vi "_Parse Text.vi"(11 "Text":string) -> (2 "Tokens":T1[](array[typedef]), 3 "Lines":string[](array[string]))   [LabVIEW 2017, in "LabVIEW-Config.lvlib" / "LabVIEW-Config.lvclass"]
uses:
  LabVIEW-Config.lvclass
  LineToken.ctl
  <userlib>/_NEVSTOP/Communicable State Machine(CSM)/Communicable State Machine.lvlib
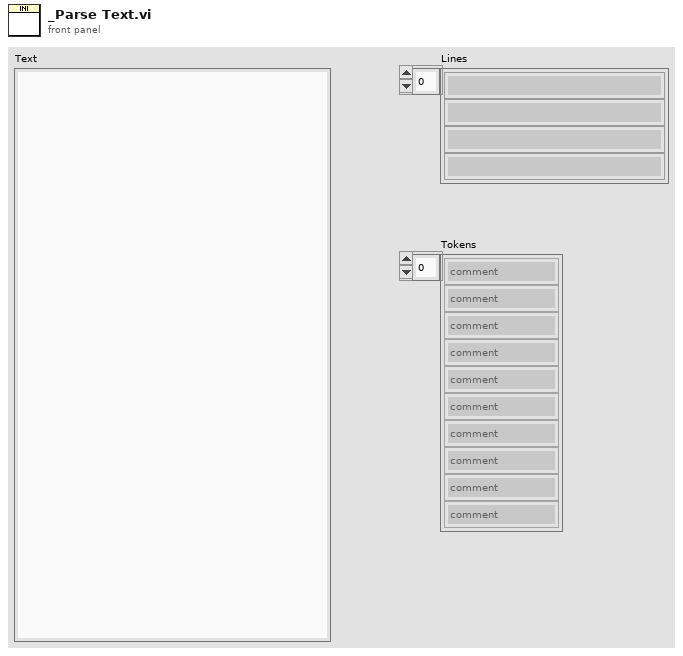
[diagram p1: front panel]
types:
  T1 = typedef "LabVIEW-Config.lvlib/LabVIEW-Config.lvclass/LineToken.ctl" = enum8{"comment", "section", "key", "more"}
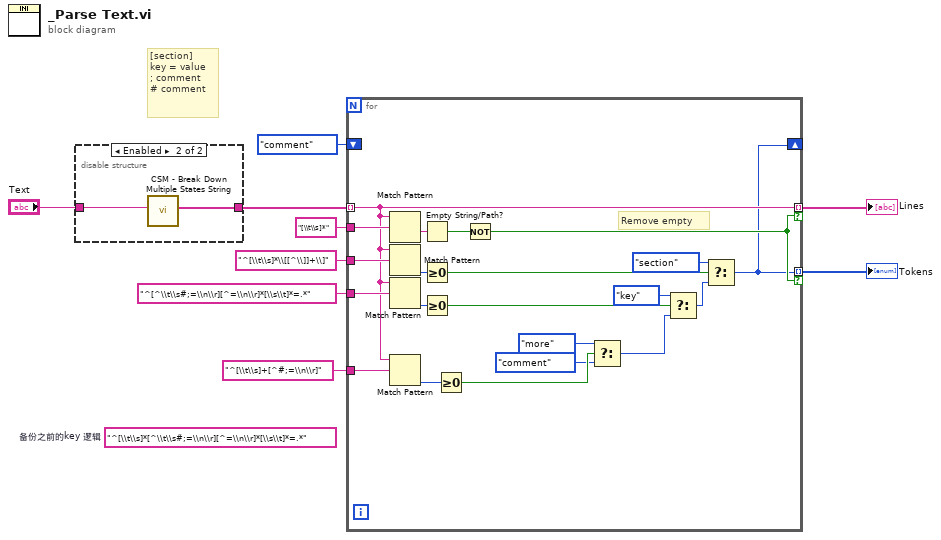
[diagram p0: block diagram]
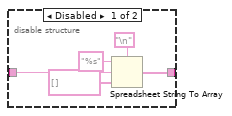
[diagram p2: hidden frame]
diagram:
  (unwired) "^[\\t\\s]*[^\\t\\s#;=\\n\\r][^=\\n\\r]*[\\s\\t]*=.*"  # 备份之前的key 逻辑
  # "[section]\nkey = value\n; comment\n# comment"
  n1 = disable-structure shown="Enabled" {
    disable-tunnel: [w14 w16] -> w7
    disable-tunnel: "Text" -> [w10 w15]
    frame Disabled {
      n2 = Spreadsheet String To Array(delimiter (Tab)="\n" ("Line Feed Constant"), format string="%s", spreadsheet string=w10, array type (2D Dbl)=string[] []) -> (array=w14:string[])
    }
    frame Enabled {
      n3 = call <userlib>:"CSM - Break Down Multiple States String.vi"("States"=w15) -> ("Multiple States"=w16:string[])  [unwired: 10 in]
    }
  }
  n4 = for {
    tunnel: w7 -> [w22] mode=indexing
    tunnel: "^[\\t\\s]*\\[[^\\]]+\\]" ("regular expression") -> [w37]
    tunnel: [w17] -> w2 mode=indexing if=w30
    tunnel: "^[^\\t\\s#;=\\n\\r][^=\\n\\r]*[\\s\\t]*=.*" ("regular expression") -> [w32]
    tunnel: "[\\t\\s]*" ("regular expression") -> [w35]
    tunnel: [w22] -> w6 mode=indexing if=w30
    tunnel: "^[\\t\\s]+[^#;=\\n\\r]" ("regular expression") -> [w23]
    shift-right: [w17] -> _
    shift-left: LineToken."comment" ("Token") -> [_]
    # "Remove empty"
    n5 = Match Pattern(string=w22, regular expression=w35) -> (after substring=w36:string)  [unwired: 1 in, 3 out]
    n6 = Match Pattern(string=w22, regular expression=w37) -> (offset past match=w34:i32)  [unwired: 1 in, 3 out]
    n7 = Match Pattern(string=w22, regular expression=w32) -> (offset past match=w33:i32)  [unwired: 1 in, 3 out]
    n8 = Match Pattern(string=w22, regular expression=w23) -> (offset past match=w24:i32)  [unwired: 1 in, 3 out]
    n9 = Empty String/Path?(string/path=w36) -> (empty?=w31:bool)
    n10 = Greater Or Equal To 0?(x=w34) -> (x >= 0?=w29:bool)
    n11 = Greater Or Equal To 0?(x=w33) -> (x >= 0?=w25:bool)
    n12 = Greater Or Equal To 0?(x=w24) -> (x >= 0?=w21:bool)
    n13 = Not(x=w31) -> (.not. x?=w30:bool)
    n14 = Select(t=LineToken."more" ("Token"), s=w21, f=LineToken."comment" ("Token")) -> (s? t:f=w18:T1)
    n15 = Select(t=LineToken."key" ("Token"), s=w25, f=w18) -> (s? t:f=w26:T1)
    n16 = Select(t=LineToken."section" ("Token"), s=w29, f=w26) -> (s? t:f=w17:T1)
  }
  "Lines" <- w6
  "Tokens" <- w2
